vi "to string.vi"(8 "error in":errorcluster, 11 "configuration in":refnum<class "TBM configuration.lvclass">) -> (0 "error out":errorcluster, 1 "data":string, 2 "version":string, 3 "configuration out":refnum<class "TBM configuration.lvclass">)   [LabVIEW 2013, in "TBM configuration.lvclass"]
doc: "Provides an interface for saving a module configuration to a file or other serialized data source. It is recommended that all children of this class store data in two sets--data required for its own initialization, and any data required for parent initialization--and that each implementation uses the <b>Call Parent Method</b> primitive to serialize parent information."
uses:
  TBM configuration.lvclass
  <vilib>/NI/CEF/CEF_TreeControl/serializable configuration/NISE_CEF_serializable configuration.lvclass
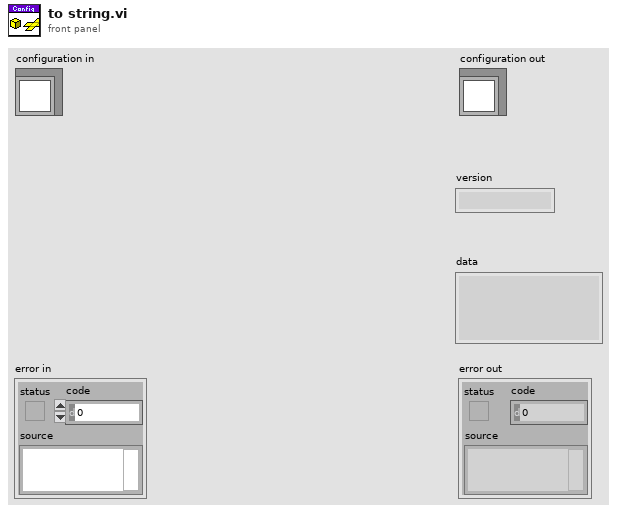
[diagram p1: front panel]
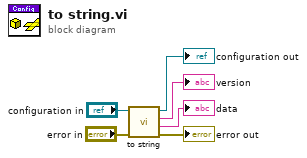
[diagram p0: block diagram]
diagram:
  n1 = call-parent "to string.vi"("error in"="error in", "configuration in"="configuration in") -> ("error out"=→"error out":errorcluster, "data"=→"data":string, "version"=→"version":string, "configuration out"=→"configuration out":refnum<class "TBM configuration.lvclass">)  [unwired: 6 in]
